vi "Reduce Samples.vi"() -> ()   [LabVIEW 2014]
panel:
  in  "Delay":dbl(knob) scale=0.0..0.1 scale format="%#_6p"
  out "Sample Mean":string[][](table) caption="Sample mean of the sine wave."
  in  "Mean":bool=TRUE caption="Enable"
  in  "stop":bool
  out "Oscilloscope":dynamicdata(graph) caption="Mean"
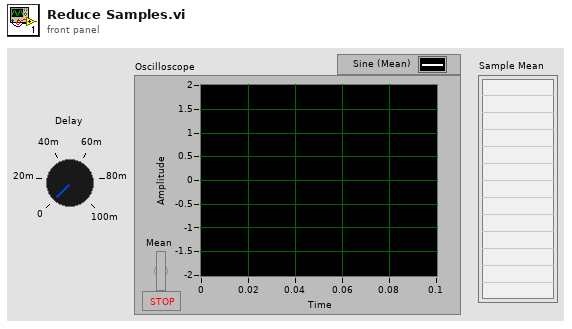
[diagram p1: front panel]
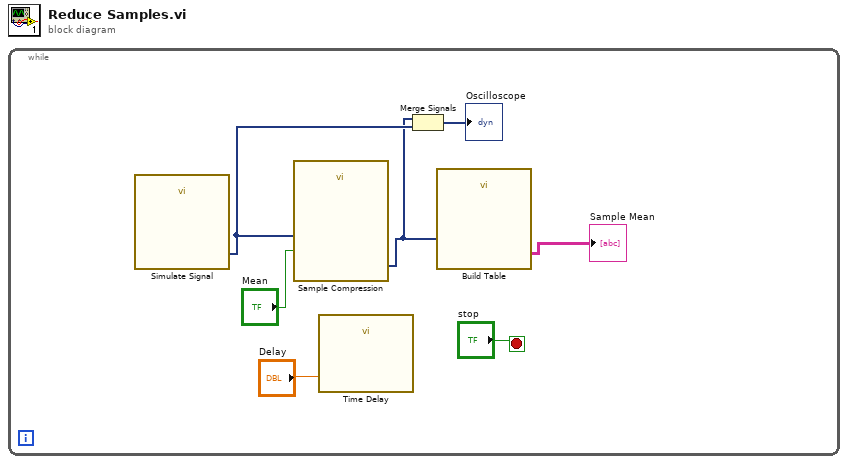
[diagram p0: block diagram]
diagram:
  n1 = while {
    stop <- "stop" stop-if-true
    n2 = call "Simulate Signal"() -> ("Sine"=w6:dynamicdata)  [unwired: 14 in, 1 out]
    n3 = call "Sample Compression"("Enable"="Mean", "Signals"=w6) -> ("Mean"=w2:dynamicdata)  [unwired: 7 in, 2 out]
    n4 = call "Time Delay"("Delay Time (s)"="Delay") -> ()  [unwired: 10 in, 1 out]
    n5 = Merge Signals(w2, w6) -> (→"Oscilloscope":dynamicdata)
    n6 = call "Build Table"("Signals"=w2) -> ("Table"=→"Sample Mean":string[][])  [unwired: 4 in, 6 out]
  }
